vi "Set Ramp To Value.vi"(0 "reference":refnum<vi>, 7 "Value":dbl) -> ()   [LabVIEW 2020]
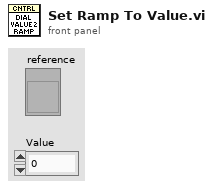
[diagram p1: front panel]
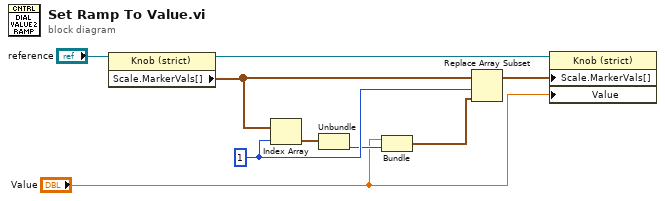
[diagram p0: block diagram]
diagram:
  w8 = 1 ("index")
  n1 = property on="Property Node" class="Knob (strict)"(reference="reference") -> (reference out=w1:refnum<vi>, "Scale.MarkerVals[]"=w9:cluster{dbl, u32}[])  [unwired: 1 in, 1 out]
  n2 = Index Array(array=w9, index=w8) -> (element=w7:cluster{dbl, u32})
  n3 = Unbundle(w7) -> (w6:u32)  [unwired: 1 out]
  n4 = Bundle("Value"="Value", w6) -> (w5:cluster{"Value":dbl, u32})  [unwired: 1 in]
  n5 = Replace Array Subset(array=w9, new element=w5, index=w8) -> (w4:cluster{dbl, u32}[])
  n6 = property on="Property Node" class="Knob (strict)"(reference=w1, "Scale.MarkerVals[]"=w4, "Value"="Value") -> ()  [unwired: 1 in, 2 out]
